vi "Init.vi"(3 "Container State":T4, 4 "Previous State":variant, 5 "Previous Version":T3) -> (2 "Current State":T1)   [LabVIEW 2020, in "3D Pie.xctl"]
uses:
  <vilib>/Math Plots/3D Math Plots/3D Pie/3D Pie XCtrl/3D Pie.xctl
  <vilib>/Math Plots/3D Math Plots/3D Pie/3D Pie XCtrl/State.ctl
  <vilib>/Math Plots/3D Math Plots/3D Pie/3D Pie/3D Pie.lvclass
  <vilib>/Math Plots/3D Math Plots/3D Plot/Action String/3DMathPlot Ctrl Act Queue.ctl
  <vilib>/Math Plots/3D Math Plots/3D Plot/Action String/3DMathPlot Ctrl Act Cluster.ctl
  <vilib>/Math Plots/3D Math Plots/3D Plot/Action String/3DMathPlot State Class.ctl
  <vilib>/_xctls/Container State.ctl
  <vilib>/_xctls/Version.ctl
  <vilib>/_xctls/XControlSupport.lvlib
panel:
  in  "Default Indicator State":T1={"3D Pie.lvclass"=refnum, "Control Ref Queue"=refnum, "Plot Width"=0, "Main Frame Color"=12369084, "Ramp Palette Color"=12369084, "Projection Palette Color"=12369084}
  in  "Default Control State":T1={"3D Pie.lvclass"=refnum, "Control Ref Queue"=refnum, "Plot Width"=0, "Main Frame Color"=12369084, "Ramp Palette Color"=12369084, "Projection Palette Color"=12369084}
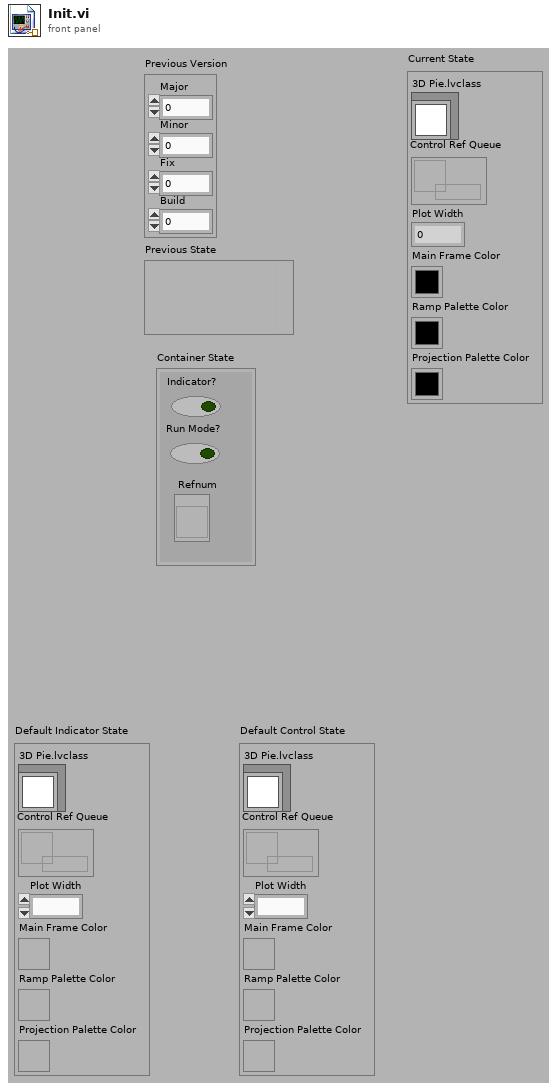
[diagram p1: front panel]
types:
  T1 = typedef "3D Pie.xctl/State.ctl" = cluster{"3D Pie.lvclass":refnum<class "3D Pie.lvclass">, "Control Ref Queue":T2, "Plot Width":u32, "Main Frame Color":u32, "Ramp Palette Color":u32, "Projection Palette Color":u32}
  T2 = typedef "3DMathPlot Ctrl Act Queue.ctl" = refnum<queue>
  T3 = typedef "XControlSupport.lvlib/Version.ctl" = cluster{"Major":u16, "Minor":u16, "Fix":u16, "Build":u16}
  T4 = typedef "XControlSupport.lvlib/Container State.ctl" = cluster{"Indicator?":bool, "Run Mode?":bool, " Refnum":refnum<vi>}
  T5 = typedef "3DMathPlot Ctrl Act Cluster.ctl" = cluster{"3D Picture Control":refnum<vi>, "Render Window Refnum":refnum<vi>, "XY Graph":refnum<vi>, "Intensity Graph":refnum<vi>, "Color Legend Palette":refnum<vi>, "Projection Palette":refnum<vi>, "XControl  Ref":refnum<vi>, "Facade Ref":refnum<vi>, "Export Image Ref":refnum<vi>, "Clear Data Flag":bool, "Display State Change Class":T6}
  T6 = typedef "3DMathPlot State Class.ctl" = enum16{"Update All Objects (Undo)", "Update Light Object Only", "Update Axis Object Only", "Update Plot Object Only", "Update Cursor Object Only", "Update Axis Plot Cursor Objects", "No Update"}
  T7 = cluster{"3D Pie.lvclass":refnum<class "3D Pie.lvclass">, "Control Ref Queue":T2}
  T8 = cluster{"3D Pie.lvclass":refnum<class "3D Pie.lvclass">, "Control Ref Queue":T2, "Plot Width":u32, "Frame Color":u32, "Frame Color":u32, "Frame Color":u32}
  T9 = cluster{"3D Pie.lvclass":refnum<class "3D Pie.lvclass">, "Control Ref Queue":T2, "Plot Width":u32}
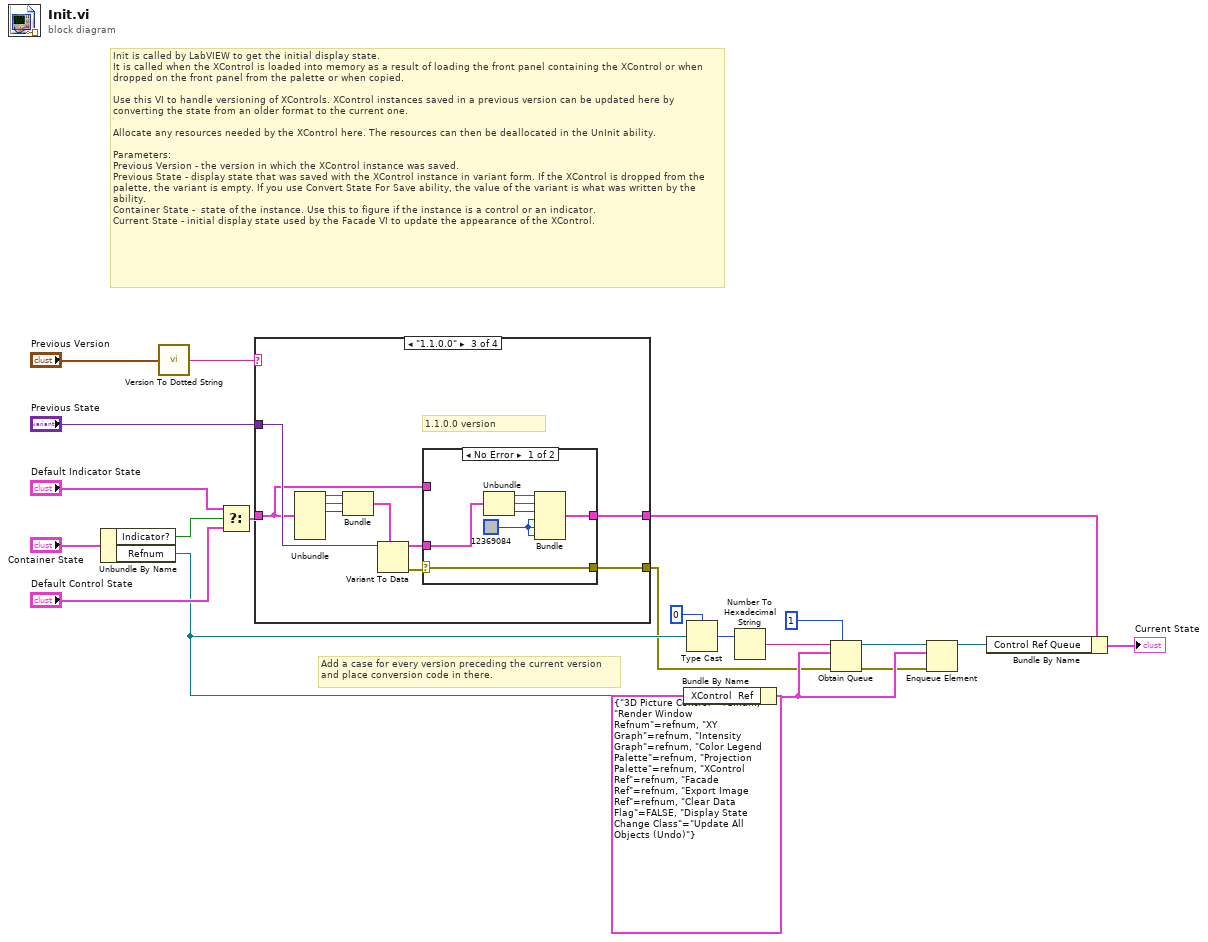
[diagram p0: block diagram]
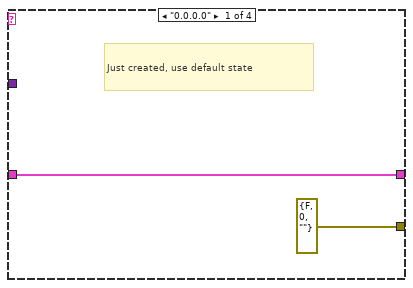
[diagram p2: hidden frame]
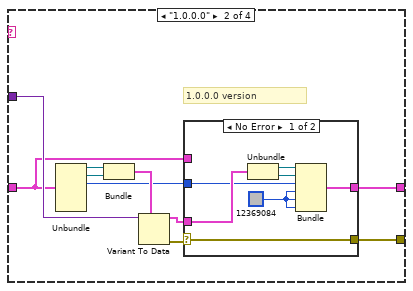
[diagram p3: hidden frame]
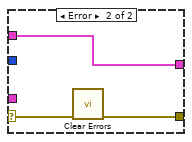
[diagram p4: hidden frame]
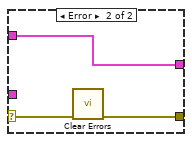
[diagram p5: hidden frame]
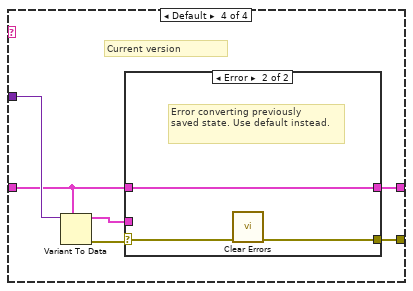
[diagram p6: hidden frame]
diagram:
  # "Init is called by LabVIEW to get the initial display state.\nIt is called when the XControl is loaded into memory as a result of loading the front panel containing the XControl or when dropped on the front panel from the palette or when copied.\n\nUse this VI to handle versioning of XControls. XControl instances saved in a previous version can be updated here by converting the state from an older format to the current one.\n\nAllocate any resources needed by the XControl here. The resources can then be deallocated in the UnInit ability.\n\nParameters:\nPrevious Version - the version in which the XControl instance was saved.\nPrevious State - display state that was saved with the XControl instance in variant form. If the XControl is dropped from the palette, the variant is empty. If you use Convert State For Save ability, the value of the variant is what was written by the ability. \nContainer State -  state of the instance. Use this to figure if the instance is a control or an indicator.\nCurrent State - initial display state used by the Facade VI to update the appearance of the XControl."
  # "Add a case for every version preceding the current version and place conversion code in there."
  n1 = Unbundle By Name("Container State") -> ("Indicator?"=w17:bool, "Refnum"=w4:refnum<vi>)
  n2 = call <vilib>:"Version To Dotted String.vi"("Version"="Previous Version") -> ("String Version"=w14:string)
  n3 = Select(t="Default Indicator State", s=w17, f="Default Control State") -> (s? t:f=w16:T1)
  n4 = case shown="\"1.1.0.0\"" w14 {
    tunnel: "Previous State" -> [_ w27 w47 w69]
    tunnel: [w23 w25 w45 w65] -> w9
    tunnel: w16 -> [w23 w26 w46 w66]
    tunnel: [errorcluster {"status"=FALSE, "code"=0, "source"=""} ("error IO") w24 w44 w64] -> w2
    frame "0.0.0.0" {
      # "Just created, use default state"
    }
    frame "1.0.0.0" {
      # "1.0.0.0 version"
      n5 = Unbundle(w26) -> ("3D Pie.lvclass"=w30:refnum<class "3D Pie.lvclass">, "Control Ref Queue"=w29:T2, "Plot Width"=w28:u32)  [unwired: 3 out]
      n6 = Bundle("3D Pie.lvclass"=w30, "Control Ref Queue"=w29) -> (w31:T7)  [unwired: 1 in]
      n7 = Variant To Data(type=w31, Variant=w27) -> (data=w32:T7, error out=w33:errorcluster)  [unwired: 1 in]
      n8 = case shown="No Error" w33 {
        selector: w33 -> [w40 w42]
        tunnel: w32 -> [w38 _]
        tunnel: [w35 w43] -> w25
        tunnel: w26 -> [_ w43]
        tunnel: [w40 w41] -> w24
        tunnel: w28 -> [w36 _]
        frame No Error {
          w34 = u32 12369084 ("Frame Color")
          n9 = Unbundle(w38) -> ("3D Pie.lvclass"=w39:refnum<class "3D Pie.lvclass">, "Control Ref Queue"=w37:T2)
          n10 = Bundle("3D Pie.lvclass"=w39, "Control Ref Queue"=w37, "Plot Width"=w36, "Frame Color"=w34, "Frame Color"=w34, "Frame Color"=w34) -> (w35:T8)  [unwired: 1 in]
        }
        frame Error {
          n11 = call <vilib>:"Clear Errors.vi"("error in (no error)"=w42) -> ("error out"=w41:errorcluster)  [unwired: 1 in, 5 out]
        }
      }
    }
    frame "1.1.0.0" {
      # "1.1.0.0 version"
      n12 = Unbundle(w46) -> ("3D Pie.lvclass"=w50:refnum<class "3D Pie.lvclass">, "Control Ref Queue"=w49:T2, "Plot Width"=w48:u32)  [unwired: 3 out]
      n13 = Bundle("3D Pie.lvclass"=w50, "Control Ref Queue"=w49, "Plot Width"=w48) -> (w51:T9)  [unwired: 1 in]
      n14 = Variant To Data(type=w51, Variant=w47) -> (data=w52:T9, error out=w53:errorcluster)  [unwired: 1 in]
      n15 = case shown="No Error" w53 {
        selector: w53 -> [w60 w62]
        tunnel: w52 -> [w58 _]
        tunnel: [w56 w63] -> w45
        tunnel: w46 -> [_ w63]
        tunnel: [w60 w61] -> w44
        frame No Error {
          w55 = u32 12369084 ("Frame Color")
          n16 = Unbundle(w58) -> ("3D Pie.lvclass"=w59:refnum<class "3D Pie.lvclass">, "Control Ref Queue"=w57:T2, "Plot Width"=w54:u32)
          n17 = Bundle("3D Pie.lvclass"=w59, "Control Ref Queue"=w57, "Plot Width"=w54, "Frame Color"=w55, "Frame Color"=w55, "Frame Color"=w55) -> (w56:T8)  [unwired: 1 in]
        }
        frame Error {
          n18 = call <vilib>:"Clear Errors.vi"("error in (no error)"=w62) -> ("error out"=w61:errorcluster)  [unwired: 1 in, 5 out]
        }
      }
    }
    frame Default {
      # "Current version"
      n19 = Variant To Data(type=w66, Variant=w69) -> (data=w67:T1, error out=w68:errorcluster)  [unwired: 1 in]
      n20 = case shown="Error" w68 {
        selector: w68 -> [w71 w73]
        tunnel: w67 -> [w70 _]
        tunnel: [w70 w74] -> w65
        tunnel: w66 -> [_ w74]
        tunnel: [w71 w72] -> w64
        frame No Error {
        }
        frame Error {
          # "Error converting previously \nsaved state. Use default instead."
          n21 = call <vilib>:"Clear Errors.vi"("error in (no error)"=w73) -> ("error out"=w72:errorcluster)  [unwired: 1 in, 5 out]
        }
      }
    }
  }
  n22 = Bundle By Name(cluster=T5 {"3D Picture Control"=refnum, "Render Window Refnum"=refnum, "XY Graph"=refnum, "Intensity Graph"=refnum, "Color Legend Palette"=refnum, "Projection Palette"=refnum, "XControl  Ref"=refnum, "Facade Ref"=refnum, "Export Image Ref"=refnum, "Clear Data Flag"=FALSE, "Display State Change Class"=enum."Update All Objects (Undo)"} ("Control Ref Cluster"), "XControl  Ref"=w4) -> (w3:T5)
  n23 = Type Cast(type=u64 0, x=w4) -> (*(type *) &x=w13:u64)
  n24 = Number To Hexadecimal String(2:w13) -> (0:w11:string)  [unwired: 1 out]
  n25 = Obtain Queue(max queue size (-1, unlimited)=1, name (unnamed)=w11, element data type=w3, error in (no error)=w2) -> (queue out=w7:refnum<queue>, error out=w1:errorcluster)  [unwired: 1 in, 1 out]
  n26 = Enqueue Element(queue=w7, element=w3, error in (no error)=w1) -> (queue out=w6:refnum<queue>)  [unwired: 3 out]
  n27 = Bundle By Name(cluster=w9, "Control Ref Queue"=w6) -> (→"Current State":T1)
